vi "二进制文件存储.vi"   [LabVIEW 2018]
types:
  T1 = enum16{"big-endian, network order", "native, host order", "little-endian"}
  T2 = enum16{"open", "replace", "create", "open or create", "replace or create", "replace or create with confirmation"}
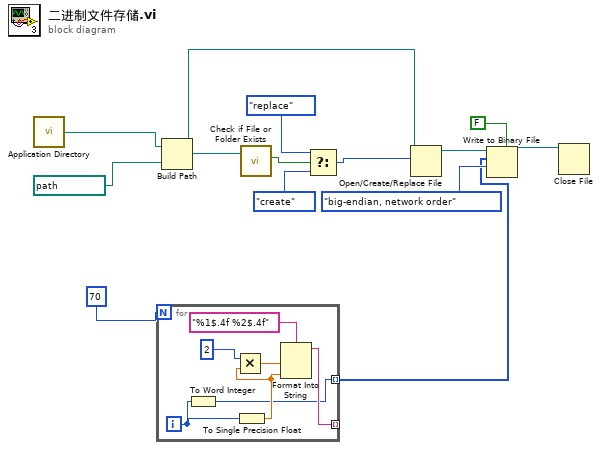
[diagram p0: block diagram]
diagram:
  n1 = call <vilib>:"Application Directory.vi"() -> ("Application Directory"=w12:path)
  n2 = for {
    N: 70 -> [_]
    tunnel: [w16] -> _ mode=indexing
    tunnel: [w14] -> w1 mode=indexing
    i -> [w15]
    n3 = To Word Integer(number=w15) -> (16bit integer=w14:i16)
    n4 = To Single Precision Float(number=w15) -> (single precision float=w20:sgl)
    n5 = Multiply(x=2, y=w20) -> (x*y=w18:sgl)
    n6 = Format Into String(format string="%1$.4f %2$.4f" ("格式字符串"), w18, w20) -> (resulting string=w16:string)  [unwired: 2 in, 1 out]
  }
  n7 = Build Path(base path=w12, name or relative path=path "二进制.dat") -> (appended path=w11:path)
  n8 = call <vilib>:"Check if File or Folder Exists.vi"("path"=w11) -> ("file or folder exists?"=w10:bool)  [unwired: 8 in, 2 out]
  n9 = Select(t=T2."replace" ("操作(0:open)"), s=w10, f=T2."create" ("操作(0:open)")) -> (s? t:f=w7:T2)
  n10 = Open/Create/Replace File(file path (use dialog)=w11, operation (0:open)=w7) -> (refnum out=w6:refnum<file>)  [unwired: 4 in, 2 out]
  n11 = Write to Binary File(file (use dialog)=w6, data=w1, 5:FALSE ("预置数组或字符串大小？ (T)"), 9:T1."big-endian, network order" ("字节顺序(0:big-endian, network order)")) -> (refnum out=w5:refnum<file>)  [unwired: 2 in, 2 out]
  n12 = Close File(refnum=w5) -> ()  [unwired: 1 in, 2 out]
